vi "Prime_Number_Detector.vi"() -> ()   [LabVIEW 2022 SP3]
panel:
  out "Prime?":bool
  in  "Number":dbl
  # "Prime Detector:\nEnter a number below to see if it is prime or not"
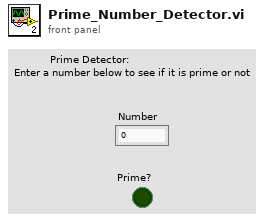
[diagram p1: front panel]
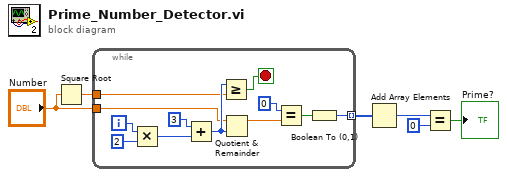
[diagram p0: block diagram]
diagram:
  n1 = Square Root(x="Number") -> (sqrt(x)=w6:dbl)
  n2 = while {
    tunnel: "Number" -> [w7]
    tunnel: w6 -> [w12]
    tunnel: [w9] -> w5 mode=indexing
    i -> [w17]
    stop <- w11 stop-if-true
    n3 = Multiply(x=w17, y=2) -> (x*y=w16:i32)
    n4 = Add(x=3, y=w16) -> (x+y=w13:i32)
    n5 = Greater Or Equal?(x=w13, y=w12) -> (x >= y?=w11:bool)
    n6 = Quotient & Remainder(x=w7, y=w13) -> (x-y*floor(x/y)=w8:dbl)  [unwired: 1 out]
    n7 = Equal?(x=0, y=w8) -> (x = y?=w10:bool)
    n8 = Boolean To (0,1)(Boolean=w10) -> (0, 1=w9:i16)
  }
  n9 = Add Array Elements(numeric array=w5) -> (sum=w4:i16)
  n10 = Equal?(x=w4, y=0) -> (x = y?=→"Prime?":bool)
